vi "XML.UpdateFromClusters.vi"(8 "error in":errorcluster, 10 "Clusters refs":refnum<vi>[](array[refnum]), 11 "XML file path":path=path "C:/Projects/TM-OS/trunk/Design/XML_HW_config2.xml") -> (0 "error out":errorcluster)   [LabVIEW 2019, in "Tools.lvlib"]
uses:
  Tools.lvlib
  <vilib>/xml/Load XML File.vi
  <vilib>/xml/NI_XML.lvlib
  <resource>/objmgr/DOMUserDefRef.rc
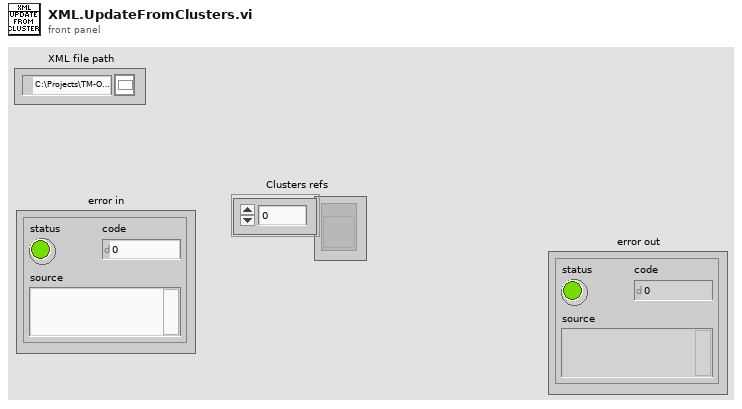
[diagram p1: front panel]
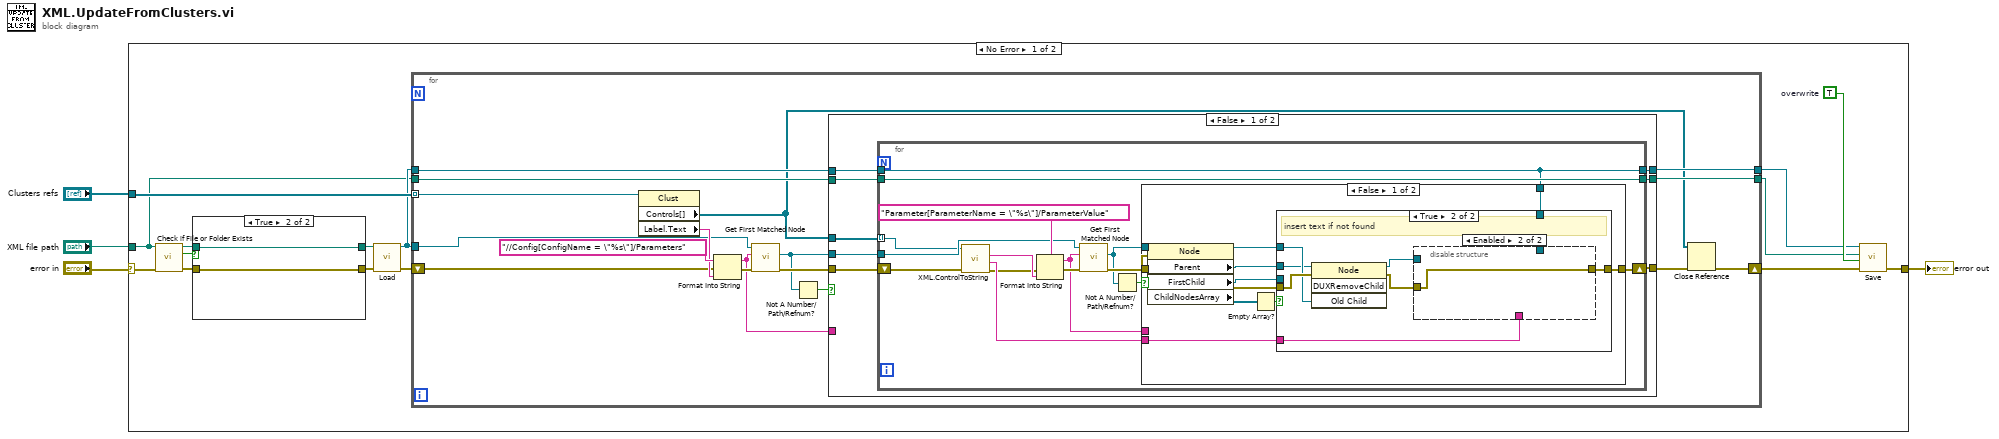
[diagram p0: block diagram]
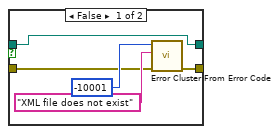
[diagram p2: hidden frame]
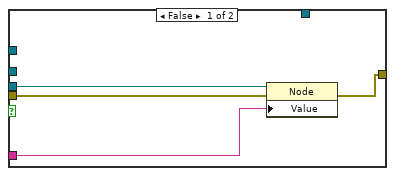
[diagram p3: hidden frame]
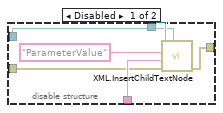
[diagram p4: hidden frame]
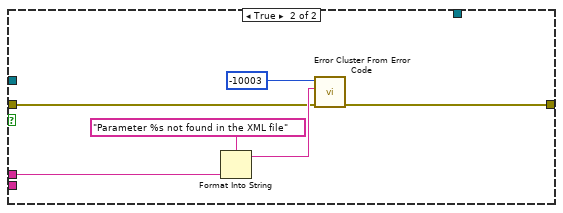
[diagram p5: hidden frame]
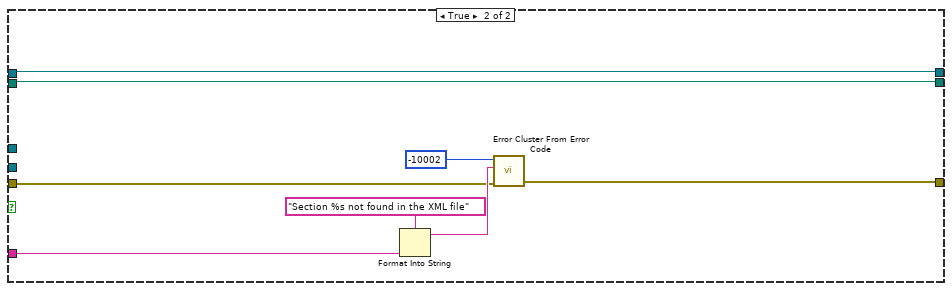
[diagram p6: hidden frame]
diagram:
  n1 = case shown="No Error" "error in" {
    selector: "error in" -> [w5 w111]
    tunnel: "Clusters refs" -> [w19 _]
    tunnel: [w16 w111] -> w4
    tunnel: "XML file path" -> [w9 _]
    frame No Error {
      w15 = TRUE  # overwrite
      n2 = call <vilib>:"Check if File or Folder Exists.vi"("error in (no error)"=w5, "path"=w9) -> ("error out"=w10:errorcluster, "file or folder exists?"=w6:bool, "dup path"=w8:path)  [unwired: 7 in]
      n3 = case shown="True" w6 {
        tunnel: [w24 w25] -> w11
        tunnel: w8 -> [w21 w26]
        tunnel: [w21 w26] -> w7
        tunnel: w10 -> [w20 w25]
        frame False {
          n4 = call <vilib>:"Error Cluster From Error Code.vi"("error in (no error)"=w20, "error message (\"\")"="XML file does not exist" ("error message (\"\")"), "error code (0)"=-10001) -> ("error out"=w24:errorcluster)  [unwired: 6 in]
        }
        frame True {
        }
      }
      n5 = call-poly <vilib>:"Load.vi"("path to XML document"=w7, "error in (no error)"=w11) -> ("DOM document out"=w14:refnum<k20>, "error out"=w18:errorcluster)  [unwired: 11 in, 1 out]
      n6 = for {
        tunnel: w19 -> [w40] mode=indexing
        shift-right: [w28] -> w17
        shift-left: w18 -> [w36]
        tunnel: w14 -> [w37]
        tunnel: [w35] -> w13
        tunnel: w14 -> [w34]
        tunnel: [w33] -> w12
        tunnel: w9 -> [w32]
        n7 = property class="Clust"(reference=w40) -> ("Controls[]"=w27:refnum<vi>[], "Label.Text"=w39:string)  [unwired: 1 in, 2 out]
        n8 = Format Into String(format string="//Config[ConfigName = \"%s\"]/Parameters" ("XPath expression"), error in=w36, w39) -> (resulting string=w29:string, error out=w41:errorcluster)  [unwired: 1 in]
        n9 = call <vilib>:"Get First Matched Node.vi"("error in (no error)"=w41, "XPath expression"=w29, "node in"=w37) -> ("error out"=w42:errorcluster, "node result"=w30:refnum<k20>)  [unwired: 6 in, 1 out]
        n10 = Not A Number/Path/Refnum?(number/path/refnum=w30) -> (NaN/Path/Refnum?=w31:bool)
        n11 = case shown="False" w31 {
          tunnel: w30 -> [w51 _]
          tunnel: w27 -> [w50 _]
          tunnel: w42 -> [w49 w107]
          tunnel: [w48 w105] -> w38
          tunnel: [w47 w104] -> w35
          tunnel: w34 -> [w46 w104]
          tunnel: [w45 w103] -> w33
          tunnel: w32 -> [w44 w103]
          tunnel: w29 -> [_ w106]
          frame False {
            n12 = for {
              tunnel: w51 -> [w65]
              tunnel: w50 -> [w60] mode=indexing
              shift-right: [w63] -> w48
              shift-left: w49 -> [w59]
              tunnel: [w55] -> w47
              tunnel: w46 -> [w55]
              tunnel: [w56] -> w45
              tunnel: w44 -> [w56]
              n13 = call "XML.ControlToString.vi"("error in"=w59, "control ref in"=w60) -> ("error out"=w58:errorcluster, "string value"=w61:string, "label"=w62:string)  [unwired: 6 in, 1 out]
              n14 = Format Into String(format string="Parameter[ParameterName = \"%s\"]/ParameterValue" ("XPath expression"), error in=w58, w62) -> (resulting string=w54:string, error out=w64:errorcluster)  [unwired: 1 in]
              n15 = call <vilib>:"Get First Matched Node.vi"("error in (no error)"=w64, "XPath expression"=w54, "node in"=w65) -> ("error out"=w57:errorcluster, "node result"=w53:refnum<k20>)  [unwired: 6 in, 1 out]
              n16 = Not A Number/Path/Refnum?(number/path/refnum=w53) -> (NaN/Path/Refnum?=w52:bool)
              n17 = case shown="False" w52 {
                tunnel: [w77 w98] -> w63
                tunnel: w61 -> [w76 _]
                tunnel: w57 -> [w75 w99]
                tunnel: w53 -> [w73 _]
                tunnel: w55 -> [w71 _]
                tunnel: w54 -> [_ w97]
                frame False {
                  n18 = property class="Node"(reference=w73, error in=w75) -> (reference out=w70:refnum<k20>, error out=w74:errorcluster, "Parent"=w68:refnum<k20>, "FirstChild"=w67:refnum<k20>, "ChildNodesArray"=w69:refnum<k20>[])
                  n19 = Empty Array?(array=w69) -> (empty?=w72:bool)
                  n20 = case shown="True" w72 {
                    tunnel: [w81 w87] -> w77
                    tunnel: w76 -> [w80 w88]
                    tunnel: w67 -> [w79 _]
                    tunnel: w74 -> [w78 w86]
                    tunnel: w70 -> [_ w84]
                    tunnel: w71 -> [_ w89]
                    tunnel: w68 -> [_ w83]
                    frame False {
                      n21 = property class="Node"(reference=w79, error in=w78, "Value"=w80) -> (error out=w81:errorcluster)  [unwired: 1 out]
                    }
                    frame True {
                      # "insert text if not found"
                      n22 = invoke class="Node" method="DUXRemoveChild"(reference=w83, error in=w86, "Old Child"=w84) -> (reference out=w82:refnum<k20>, error out=w85:errorcluster)  [unwired: 1 in, 2 out]
                      n23 = disable-structure shown="Enabled" {
                        disable-tunnel: w89 -> [w95 _]
                        disable-tunnel: w88 -> [w93 _]
                        disable-tunnel: [w92 w96] -> w87
                        disable-tunnel: w85 -> [w91 w96]
                        disable-tunnel: w82 -> [w90 _]
                        frame Disabled {
                          n24 = call "XML.InsertChildTextNode.vi"("parent"=w90, "error in"=w91, "text"=w93, "name"="ParameterValue", "doc"=w95) -> ("error out"=w92:errorcluster)  [unwired: 5 in, 1 out]
                        }
                        frame Enabled {
                        }
                      }
                    }
                  }
                }
                frame True {
                  n25 = Format Into String(format string="Parameter %s not found in the XML file", w97) -> (resulting string=w102:string)  [unwired: 2 in, 1 out]
                  n26 = call <vilib>:"Error Cluster From Error Code.vi"("error in (no error)"=w99, "error message (\"\")"=w102, "error code (0)"=-10003) -> ("error out"=w98:errorcluster)  [unwired: 6 in]
                }
              }
            }
          }
          frame True {
            n27 = Format Into String(format string="Section %s not found in the XML file", w106) -> (resulting string=w108:string)  [unwired: 2 in, 1 out]
            n28 = call <vilib>:"Error Cluster From Error Code.vi"("error in (no error)"=w107, "error message (\"\")"=w108, "error code (0)"=-10002) -> ("error out"=w105:errorcluster)  [unwired: 6 in]
          }
        }
        n29 = Close Reference(reference=w27, error in (no error)=w38) -> (error out=w28:errorcluster)
      }
      n30 = call <vilib>:"Save.vi"("error in (no error)"=w17, "overwrite file (True)"=w15, "XML file path"=w12, "DOM document in"=w13) -> ("error out"=w16:errorcluster)  [unwired: 5 in, 2 out]
    }
    frame Error {
    }
  }
  "error out" <- w4
